vi "PRACTICA 5.vi"() -> ()   [LabVIEW 2017]
panel:
  out "x > 0?":bool
  in  "stop":bool
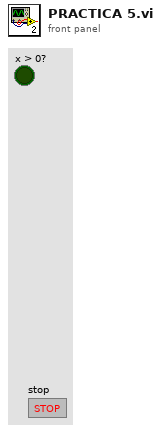
[diagram p1: front panel]
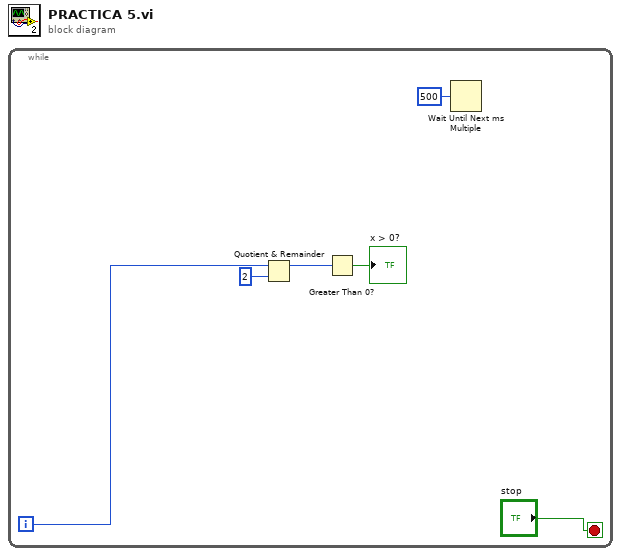
[diagram p0: block diagram]
diagram:
  n1 = while {
    i -> [w4]
    stop <- "stop" stop-if-true
    n2 = Quotient & Remainder(x=w4, y=2) -> (x-y*floor(x/y)=w2:i32)  [unwired: 1 out]
    n3 = Greater Than 0?(x=w2) -> (x > 0?=→"x > 0?":bool)
    n4 = Wait Until Next ms Multiple(millisecond multiple=u32 500) -> ()  [unwired: 1 out]
  }
